vi "BuildFarm Directory.vi"() -> (0 "BuildFarm Directory":path)   [LabVIEW 2017]
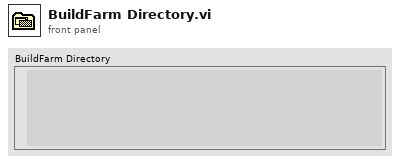
[diagram p1: front panel]
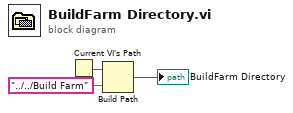
[diagram p0: block diagram]
diagram:
  n1 = Current VI's Path() -> (path=w2:path)
  n2 = Build Path(base path=w2, name or relative path="../../Build Farm") -> (appended path=→"BuildFarm Directory":path)
